vi "CmdConsole.Read STDOUT Queue.vi"(10 "QName":string="StdOut", 11 "StdOut Ctrl":refnum<vi>) -> ()   [LabVIEW 2018]
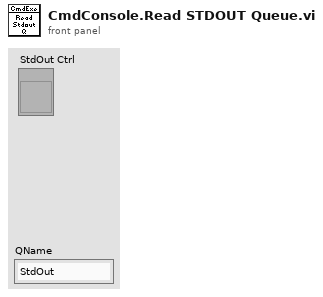
[diagram p1: front panel]
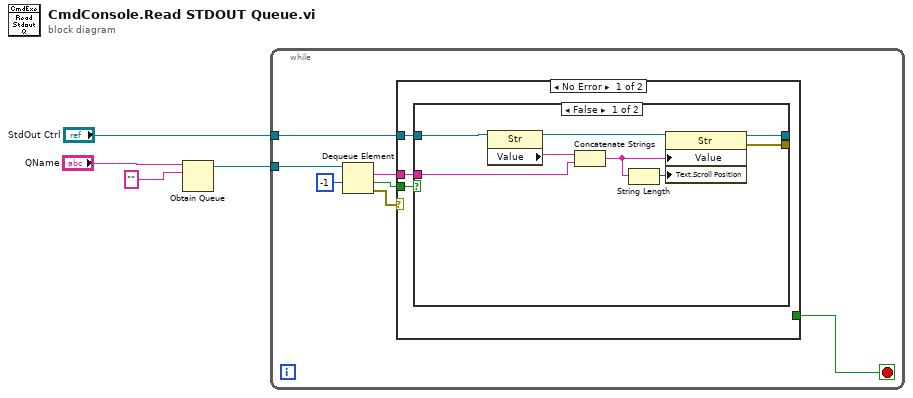
[diagram p0: block diagram]
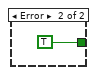
[diagram p3: hidden frame]
diagram:
  n1 = Obtain Queue(name (unnamed)="QName", element data type="") -> (queue out=w2:refnum<queue>)  [unwired: 3 in, 2 out]
  n2 = while {
    tunnel: w2 -> [w11]
    tunnel: "StdOut Ctrl" -> [w10]
    stop <- w7 stop-if-true
    n3 = Dequeue Element(queue=w11, timeout in ms (-1)=-1) -> (element=w8:string, timed out?=w5:bool, error out=w9:errorcluster)  [unwired: 1 in, 1 out]
    n4 = case shown="No Error" w9 {
      tunnel: w10 -> [w14 _]
      tunnel: w8 -> [w13 _]
      tunnel: [_ TRUE] -> w7
      tunnel: w5 -> [w12 _]
      frame No Error {
        n5 = case shown="False" w12 {
          tunnel: w14 -> [w21 _]
          tunnel: w13 -> [w15 _]
          tunnel: [w17 _] -> _
          tunnel: [w16 _] -> _
          frame False {
            n6 = property class="Str"(reference=w21) -> (reference out=w18:refnum<vi>, "Value"=w19:string)  [unwired: 1 in, 1 out]
            n7 = Concatenate Strings(w19, w15) -> (w20:string)
            n8 = String Length(string=w20) -> (length=w22:i32)
            n9 = property class="Str"(reference=w18, "Value"=w20, "Text.Scroll Position"=w22) -> (reference out=w17:refnum<vi>, error out=w16:errorcluster)  [unwired: 1 in]
          }
          frame True {
          }
        }
      }
      frame Error {
      }
    }
  }
